vi "Configure Integration.vi"(8 "error in (no error)":errorcluster, 9 "Integration Time (10 PLCs)":dbl(ring)=10.0 items=["0.02"=0.02, "0.2"=0.2, "1"=1.0, "10"=10.0, "100"=100.0], 10 "Function (0: DC Voltage)":u16(ring) items=["DC Voltage", "AC Voltage", "2 - Wire Resistance", "4 - Wire Resistance", "DC Current", "AC Current", "Frequency", "Period", "Continuity", "Diode Checking", "Temperature", "Capacitance"], 11 "VISA resource name":refnum<visa-resource-name>) -> (0 "error out":errorcluster, 3 "VISA resource name out":refnum<visa-resource-name>)   [LabVIEW 2010, in "Fluke 884X Series.lvlib"]
doc: "Configures the amount of time the analog to digital converter samples a signal. A longer integration time leads to a higher resolution. Auto Ranging must be disabled for these settings to apply.\n\n<b>Applicable Functions:</b>\nAll models:\n DC Voltage\n 2-Wire Resistance\n 4-Wire Resistance\n DC Current\n Temperature\n\n<B>Note1:</B>\n\nChanging the integration time may change the resolution configured in the <B>Configure Measurement VI</B>.\n\n<B>Note2:</B>\n\nFluke 8845A does not support Temperature or Capacitance configurations or measurements."
uses:
  <instrlib>/Fluke 884X Series/Fluke 884X Series.lvlib
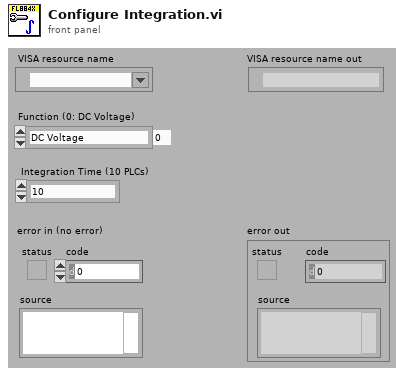
[diagram p1: front panel]
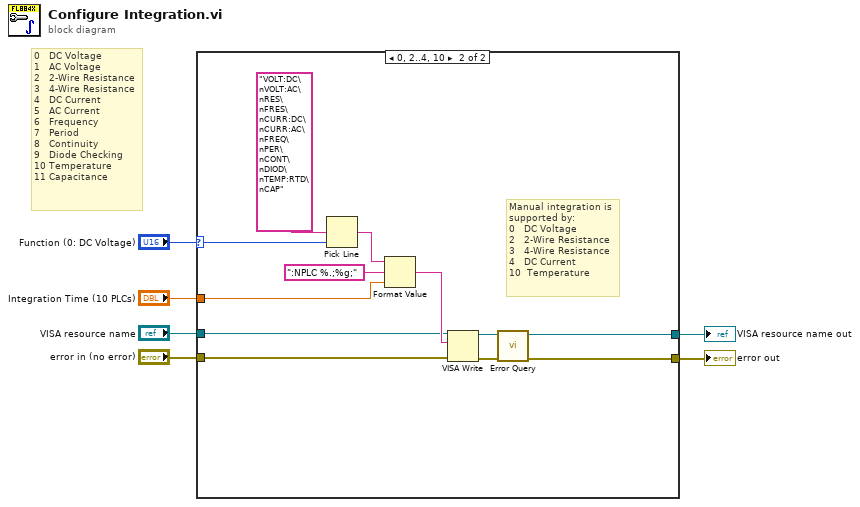
[diagram p0: block diagram]
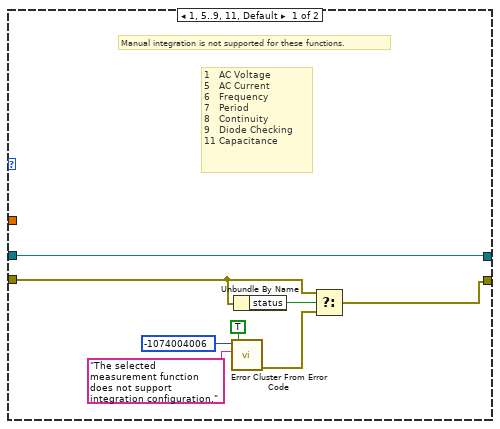
[diagram p2: hidden frame]
diagram:
  # "0   DC Voltage\n1   AC Voltage\n2   2-Wire Resistance\n3   4-Wire Resistance\n4   DC Current\n5   AC Current\n6   Frequency\n7   Period\n8   Continuity\n9   Diode Checking\n10 Temperature\n11 Capacitance"
  n1 = case shown="0, 2..4, 10" "Function (0: DC Voltage)" {
    selector: "Function (0: DC Voltage)" -> [_ w19]
    tunnel: "VISA resource name" -> [w14 w17]
    tunnel: "error in (no error)" -> [w9 w16]
    tunnel: [w14 w22] -> w3
    tunnel: [w7 w21] -> w2
    tunnel: "Integration Time (10 PLCs)" -> [_ w20]
    frame 1, 5..9, 11, Default {
      # "1   AC Voltage\n5   AC Current\n6   Frequency\n7   Period\n8   Continuity\n9   Diode Checking\n11 Capacitance"
      # "Manual integration is not supported for these functions."
      n2 = call <vilib>:"Error Cluster From Error Code.vi"("show call chain? (False)"=TRUE, "error message (\"\")"="The selected measurement function does not support integration configuration." ("Source (VI Name)"), "error code (0)"=-1074004006 ("Code")) -> ("error out"=w8:errorcluster)  [unwired: 6 in]
      n3 = Unbundle By Name(w9) -> ("status"=w10:bool)
      n4 = Select(t=w9, s=w10, f=w8) -> (s? t:f=w7:errorcluster)
    }
    frame 0, 2..4, 10 {
      # "Manual integration is  supported by:\n0   DC Voltage\n2   2-Wire Resistance\n3   4-Wire Resistance\n4   DC Current\n10  Temperature"
      n5 = Pick Line(multi-line string="VOLT:DC\nVOLT:AC\nRES\nFRES\nCURR:DC\nCURR:AC\nFREQ\nPER\nCONT\nDIOD\nTEMP:RTD\nCAP", line index=w19) -> (output string=w23:string)  [unwired: 1 in]
      n6 = Format Value(string ("")=w23, format string=":NPLC %.;%g;", value (0)=w20) -> (output string=w18:string)
      n7 = VISA Write(VISA resource name=w17, write buffer=w18, error in (no error)=w16) -> (VISA resource name out=w26:refnum<visa-resource-name>, error out=w25:errorcluster)  [unwired: 1 out]
      n8 = call <instrlib>:"Error Query.vi"("error in (no error)"=w25, "VISA resource name"=w26) -> ("error out"=w21:errorcluster, "VISA resource name out"=w22:refnum<visa-resource-name>)  [unwired: 6 in, 2 out]
    }
  }
  "error out" <- w2
  "VISA resource name out" <- w3
